vi "Update Count.vi"(8 "error in (no error)":errorcluster, 10 "Count":u64, 11 "Work in":refnum<class "Work.lvclass">) -> (0 "error out":errorcluster, 3 "Work out":refnum<class "Work.lvclass">)   [LabVIEW 2024, in "Chef State.lvlib" / "Work.lvclass"]
uses:
  Work.lvclass
  <vilib>/ActorFramework/Actor/Actor.lvclass/Actor.ctl
  Chef UI Logic/Chef UI Logic Messages/Update Count Msg/Update Count Msg.lvclass/Update Count Msg.ctl
  <vilib>/ActorFramework/Message Enqueuer/Message Enqueuer.lvclass/Message Enqueuer.ctl
  <vilib>/ActorFramework/Message Enqueuer/Enqueue.vi
  Chef UI Logic/Chef UI Logic Messages/Update Count Msg/Update Count Msg.lvclass
  C:/Program Files/National Instruments/LabVIEW 2024/vi.lib/ActorFramework/Message/Message.lvclass
  <vilib>/ActorFramework/Message Priority Queue/Priority Enqueue.vi
  Work.lvclass/Work.ctl
  <vilib>/ActorFramework/Actor/Actor.lvclass
  C:/Users/burakkorkmaz/Desktop/PROJE/actor-state-machine/Chef State/Chef State/Chef State.lvclass
  C:/Program Files/National Instruments/LabVIEW 2024/vi.lib/NI/Actors/State Actor/State Actor/State Actor.lvclass
  C:/Program Files/National Instruments/LabVIEW 2024/vi.lib/ActorFramework/Actor/Actor.lvclass
  C:/Users/burakkorkmaz/Desktop/PROJE/actor-state-machine/Chef State/Work/Work.lvclass
  C:/Users/burakkorkmaz/Desktop/PROJE/actor-state-machine/Chef State Logic/Work Logic/Work Logic.lvclass
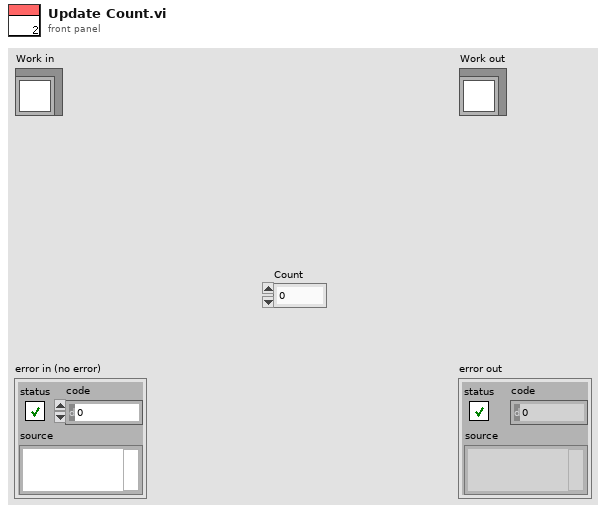
[diagram p1: front panel]
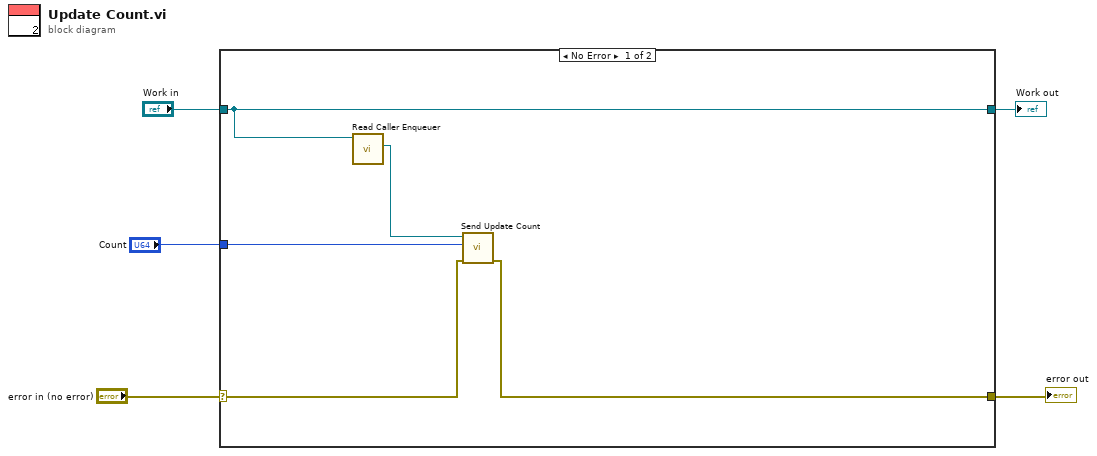
[diagram p0: block diagram]
diagram:
  n1 = case shown="No Error" "error in (no error)" {
    selector: "error in (no error)" -> [w9 w11]
    tunnel: [w8 w11] -> w4
    tunnel: "Work in" -> [w7 w12]
    tunnel: [w7 w12] -> w2
    tunnel: "Count" -> [w10 _]
    frame No Error {
      n2 = call <vilib>:"Read Caller Enqueuer.vi"("Actor"=w7) -> ("Caller Enqueuer"=w6:refnum<class "Message Enqueuer.lvclass">)  [unwired: 10 in]
      n3 = call "Send Update Count.vi"("error in (no error)"=w9, "Count"=w10, "Message Enqueuer"=w6) -> ("error out"=w8:errorcluster)  [unwired: 7 in, 1 out]
    }
    frame Error {
    }
  }
  "error out" <- w4
  "Work out" <- w2
